vi "config_read.vi"(8 "error in (no error)":errorcluster) -> (0 "error out":errorcluster, 3 "configuration":T1)   [LabVIEW 2015, in "lv-recipe-machine.lvlib"]
doc: "This VI can be used to read the most recent configuration stored in the shared data notifier. It can be accessed publically and is vulnerable to read race conditions although the configuration should only change if the module is initialized or re-initialized."
uses:
  lv-recipe-machine.lvlib
  _controls/configuration.ctl
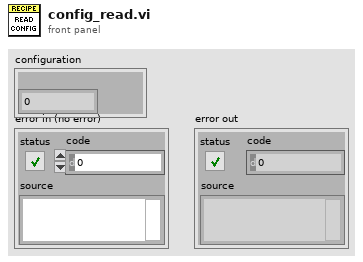
[diagram p1: front panel]
types:
  T1 = typedef "lv-recipe-machine.lvlib/configuration.ctl" = cluster{"change_in_timeout_ms":i32}
  T2 = typedef "lv-recipe-machine.lvlib/references.ctl" = cluster{"semaphore":T3, "input_queue":refnum<queue>, "output_queue":refnum<queue>, "transition_queue":refnum<queue>, "data_dvr":refnum<data-value>, "stop_notifier":refnum<notifier>, "change_in_event":refnum<user-event>, "change_out_event":refnum<user-event>, "status_event":refnum<user-event>}
  T3 = typedef "Semaphore RefNum" = refnum<k1>
  T4 = typedef "lv-recipe-machine.lvlib/data.ctl" = cluster{"configuration":T1, "working":cluster{"recipe_data":T5}}
  T5 = typedef "lv-recipe-machine.lvlib/recipe_data.ctl" = cluster{"mode":T6, "manual_state":T7, "automatic_state":T8, "previous_automatic_state":T8, "error":errorcluster, "timer []":T9[], "manual":cluster{"step_action":string, "data":variant, "actions":variant}, "automatic":cluster{"data":variant, "steps":variant, "criteria":variant, "transition":string, "index":i32, "recipe []":T10[]}}
  T6 = typedef "lv-recipe-machine.lvlib/mode.ctl" = enum16{"<mode>", "manual", "automatic", "<null>"}
  T7 = typedef "lv-recipe-machine.lvlib/manual_state.ctl" = enum16{"<manual_state>", "failed", "action", "running", "idle", "<null>"}
  T8 = typedef "lv-recipe-machine.lvlib/automatic_state.ctl" = enum16{"<automatic_state>", "failed", "idle", "running", "paused", "stopped", "<null>"}
  T9 = typedef "lv-recipe-machine.lvlib/timer.ctl" = cluster{"elapsed_time":dbl, "previous_time":dbl}
  T10 = typedef "lv-recipe-machine.lvlib/recipe_step.ctl" = cluster{"step":string, "data":variant}
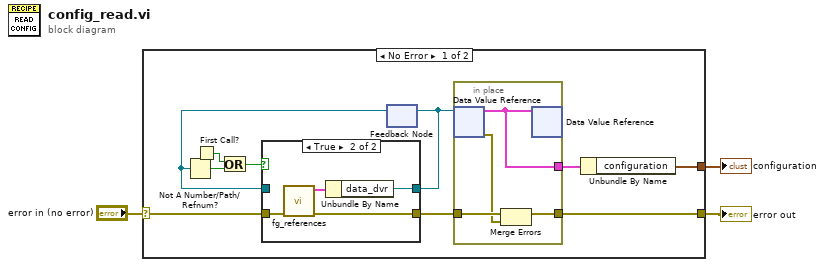
[diagram p0: block diagram]
diagram:
  n1 = case shown="No Error" "error in (no error)" {
    selector: "error in (no error)" -> [w5 w24]
    tunnel: [w12 w24] -> w2
    tunnel: [w13 _] -> w1
    frame No Error {
      n2 = First Call?() -> (First Call?: T/F=w9:bool)
      n3 = feedback #1() -> (w8:refnum<data-value>)  [unwired: 1 in]
      n4 = Not A Number/Path/Refnum?(number/path/refnum=w8) -> (NaN/Path/Refnum?=w10:bool)
      n5 = Or(x=w9, y=w10) -> (x .or. y?=w7:bool)
      n6 = case shown="True" w7 {
        tunnel: w5 -> [w14 w19]
        tunnel: [w14 w18] -> w4
        tunnel: [w15 w16] -> w6
        tunnel: w8 -> [w15 _]
        frame False {
        }
        frame True {
          n7 = call "fg_references.vi"("error in (no error)"=w19) -> ("error out"=w18:errorcluster, "references out"=w17:T2)  [unwired: 9 in]
          n8 = Unbundle By Name(w17) -> ("data_dvr"=w16:refnum<data-value>)
        }
      }
      n9 = feedback-in #1(w6) -> ()
      n10 = in-place {
        in-place-border: w4 -> [w23]
        in-place-border: [w21] -> w11
        in-place-border: [w20] -> w12
        n11 = in-place-dvr #2(w6) -> (w21:T4, w22:errorcluster)
        n12 = Merge Errors(w23, w22) -> (w20:errorcluster)
        n13 = in-place-dvr #2(w21) -> ()  [unwired: 2 out]
      }
      n14 = Unbundle By Name(w11) -> ("configuration"=w13:T1)
    }
    frame Error {
    }
  }
  "error out" <- w2
  "configuration" <- w1
